vi "output.vi"(8 "error in":errorcluster, 10 "data table in":T1, 11 "EIP Tags Runtime in":refnum<class "EIP Tags Runtime.lvclass">) -> (0 "error out":errorcluster, 2 "data table out":T1, 3 "EIP Tags Runtime out":refnum<class "EIP Tags Runtime.lvclass">)   [LabVIEW 2013, in "EIP Tags Runtime.lvclass"]
doc: "Provides an interface for writing data to a module at runtime. While this interface performs no operations, a child should provide an override which may write to any open sessions, references, or interfaces."
uses:
  EIP Tags Runtime.lvclass
  <vilib>/NI/Tag Bus/table/data table.ctl
  EIP Tags Runtime.lvclass/EIP Tags Runtime.ctl
  <vilib>/NI/Tag Bus/table/data polymorphs/read many/read I8s.vi
  <vilib>/NI/Tag Bus/table/data polymorphs/read one/read Array of I8.vi
  <vilib>/NI/Tag Bus/table/data polymorphs/read many/read I16s.vi
  <vilib>/NI/Tag Bus/table/data polymorphs/read one/read Array of I16.vi
  <vilib>/NI/Tag Bus/table/data polymorphs/read many/read I32s.vi
  <vilib>/NI/Tag Bus/table/data polymorphs/read one/read Array of I32.vi
  <vilib>/NI/Tag Bus/table/data polymorphs/read many/read Singles.vi
  <vilib>/NI/Tag Bus/table/data polymorphs/read one/read Array of Single.vi
  <vilib>/NI/Tag Bus/table/data polymorphs/read many/read Booleans.vi
  <vilib>/NI/Tag Bus/table/data polymorphs/read one/read Array of Boolean.vi
  <vilib>/NI/Tag Bus/table/data polymorphs/read one/read String.vi
  <vilib>/ethernetip/ethernetip.llb/EthernetIP Tag Write SINT.vi
  <vilib>/ethernetip/ethernetip.llb/EthernetIP Tag Write INT.vi
  <vilib>/ethernetip/ethernetip.llb/EthernetIP Tag Write DINT.vi
  <vilib>/ethernetip/ethernetip.llb/EthernetIP Tag Write REAL.vi
  <vilib>/ethernetip/ethernetip.llb/EthernetIP Tag Write BOOL.vi
  <vilib>/ethernetip/ethernetip.llb/EthernetIP Tag Write STRING.vi
  <vilib>/NI/Tag Bus/table/data table.lvlib
  <vilib>/ethernetip/ethernetip.lvlib
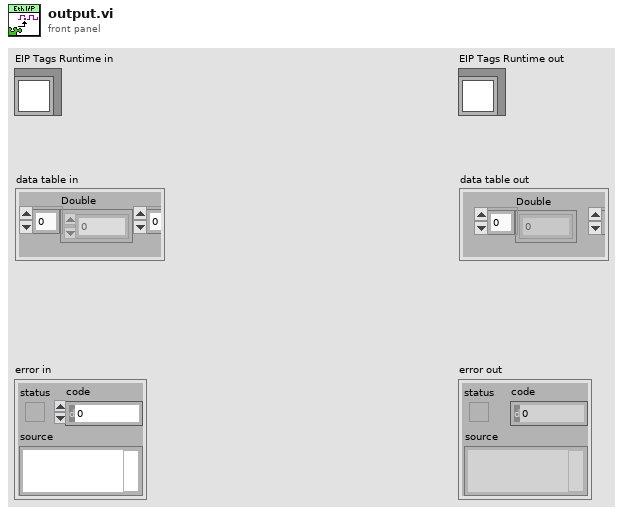
[diagram p1: front panel]
types:
  T1 = typedef "tag bus.lvlib/data table.lvlib/data table.ctl" = cluster{"Double":dbl[], "Single":sgl[], "I64":i64[], "I32":i32[], "I16":i16[], "I8":i8[], "U64":u64[], "U32":u32[], "U16":u16[], "U8":u8[], "Boolean":bool[], "String":string[], "Array of Double":cluster{"DBL Array":dbl[]}[], "Array of Single":cluster{"SGL Array":sgl[]}[], "Array of I64":cluster{"I64 Array":i64[]}[], "Array of I32":cluster{"I32 Array":i32[]}[], "Array of I16":cluster{"I16 Array":i16[]}[], "Array of I8":cluster{"I8 Array":i8[]}[], "Array of U64":cluster{"U64 Array":u64[]}[], "Array of U32":cluster{"U32 Array":u32[]}[], "Array of U16":cluster{"U16 Array":u16[]}[], "Array of U8":cluster{"U8 Array":u8[]}[], "Array of Boolean":cluster{"Boolean Array":bool[]}[], "Array of String":cluster{"String Array":string[]}[]}
  T2 = typedef "ethernetip.lvlib/ethernetip.ctl" = refnum<k21>
  T3 = typedef "EIP Tags Runtime.lvclass/eip tag spec.ctl" = cluster{"eip tag types":T4, "Network Path":string, "Tag Name":string, "Number of Elements":u32, "data indices":i32[], "tag bus indices":i32[], "array tbtag":bool}
  T4 = typedef "EIP Tags Configuration.lvclass/eip tag types.ctl" = enum16{"SINT", "INT", "DINT", "REAL", "BOOL", "STRING"}
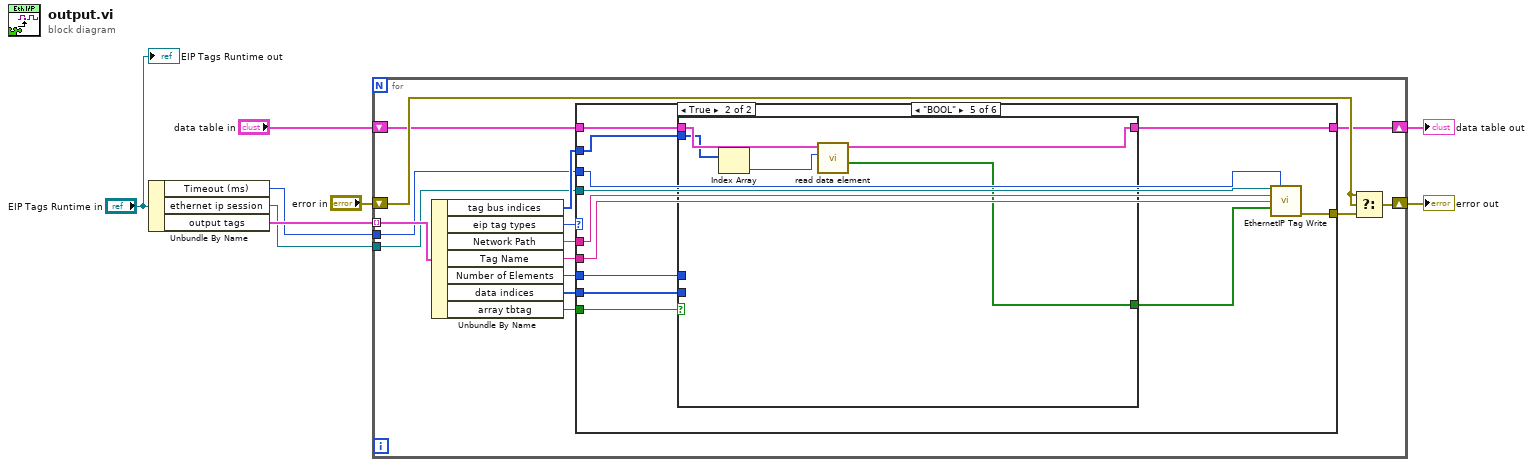
[diagram p0: block diagram]
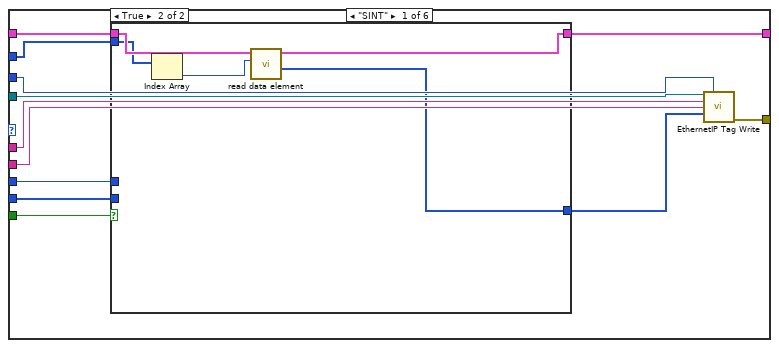
[diagram p2: hidden frame]
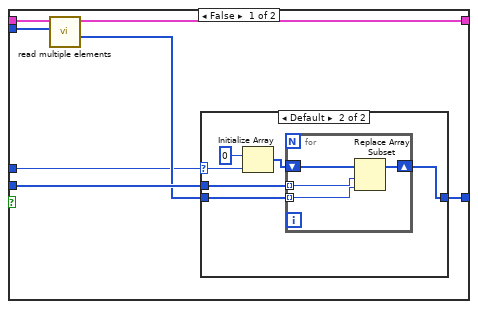
[diagram p3: hidden frame]
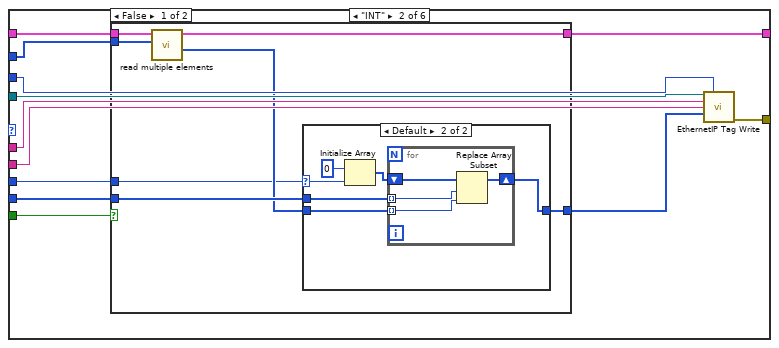
[diagram p5: hidden frame]
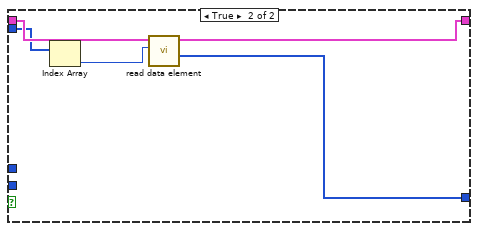
[diagram p7: hidden frame]
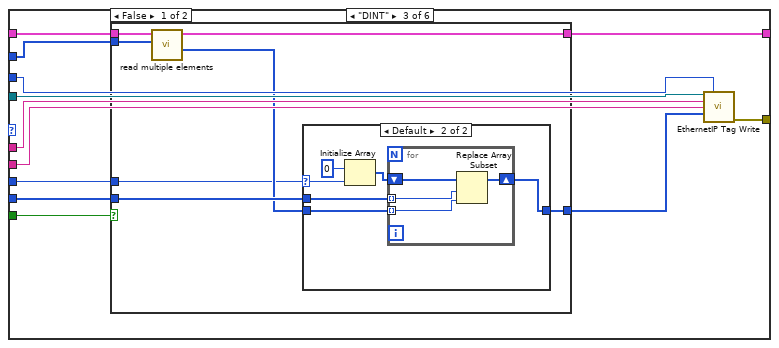
[diagram p8: hidden frame]
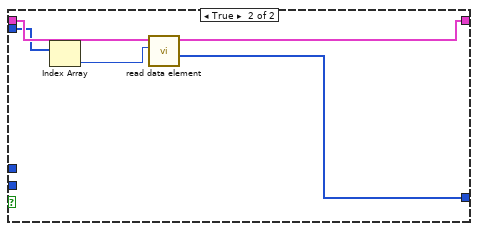
[diagram p10: hidden frame]
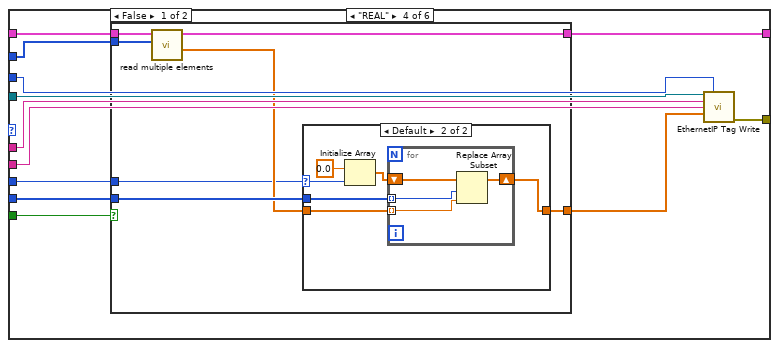
[diagram p11: hidden frame]
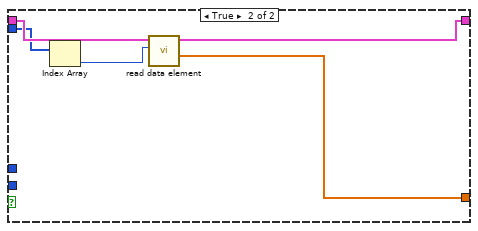
[diagram p13: hidden frame]
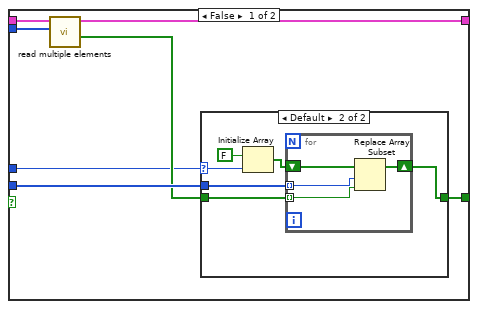
[diagram p14: hidden frame]
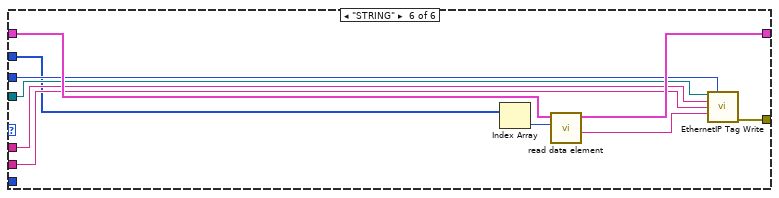
[diagram p16: hidden frame]
diagram:
  n1 = Unbundle By Name("EIP Tags Runtime in") -> ("Timeout (ms)"=w1:i32, "ethernet ip session"=w2:T2, "output tags"=w3:T3[])
  n2 = for {
    shift-right: [w22] -> w7
    shift-left: "error in" -> [w23]
    shift-right: [w19] -> w5
    shift-left: "data table in" -> [w18]
    tunnel: w3 -> [w21] mode=indexing
    tunnel: w2 -> [w16]
    tunnel: w1 -> [w15]
    n3 = Unbundle By Name(w21) -> ("tag bus indices"=w17:i32[], "eip tag types"=w20:T4, "Network Path"=w14:string, "Tag Name"=w13:string, "Number of Elements"=w12:u32, "data indices"=w10:i32[], "array tbtag"=w9:bool)
    n4 = case shown="\"BOOL\"" w20 {
      tunnel: [w34 w69 w104 w139 w174 w207] -> w19
      tunnel: w18 -> [w35 w70 w105 w140 w175 w208]
      tunnel: w17 -> [w33 w68 w103 w138 w173 w201]
      tunnel: w16 -> [w32 w67 w102 w137 w172 w206]
      tunnel: w15 -> [w31 w66 w101 w136 w171 w205]
      tunnel: w14 -> [w30 w65 w100 w135 w170 w204]
      tunnel: w13 -> [w29 w64 w99 w134 w169 w203]
      tunnel: w12 -> [w25 w60 w95 w130 w165 _]
      tunnel: [w27 w62 w97 w132 w167 w202] -> w11
      tunnel: w10 -> [w26 w61 w96 w131 w166 _]
      tunnel: w9 -> [w24 w59 w94 w129 w164 _]
      frame "SINT" {
        n5 = case shown="True" w24 {
          tunnel: w35 -> [w42 w58]
          tunnel: [w41 w54] -> w34
          tunnel: w33 -> [w40 w57]
          tunnel: [w39 w55] -> w28
          tunnel: w26 -> [w38 _]
          tunnel: w25 -> [w36 _]
          frame False {
            n6 = call-poly <vilib>:"read multiple elements.vi"("indices"=w40, "data table in"=w42) -> ("values"=w37:i8[], "data table out"=w41:T1)  [unwired: 8 in]
            n7 = case shown="Default" w36 {
              selector: w36 -> [_ w44]
              tunnel: [w43 w47] -> w39
              tunnel: w38 -> [_ w46]
              tunnel: w37 -> [w43 w45]
              frame 1 {
              }
              frame Default {
                n8 = Initialize Array(i8 0, w44) -> (w48:i8[])
                n9 = for {
                  shift-right: [w52] -> w47
                  shift-left: w48 -> [w53]
                  tunnel: w46 -> [w51] mode=indexing
                  tunnel: w45 -> [w50] mode=indexing
                  n10 = Replace Array Subset(array=w53, new element=w50, index=w51) -> (w52:i8[])
                }
              }
            }
          }
          frame True {
            n11 = Index Array(array=w57) -> (element=w56:i32)  [unwired: 1 in]
            n12 = call-poly <vilib>:"read data element.vi"("index"=w56, "data table in"=w58) -> ("value"=w55:i8[], "data table out"=w54:T1)  [unwired: 8 in]
          }
        }
        n13 = call-poly <vilib>:"EthernetIP Tag Write.vi"("Session in"=w32, "Timeout (ms)"=w31, "Network Path"=w30, "Tag Name"=w29, "Data"=w28) -> ("error out"=w27:errorcluster)  [unwired: 9 in, 1 out]
      }
      frame "INT" {
        n14 = case shown="False" w59 {
          tunnel: w70 -> [w77 w93]
          tunnel: [w76 w89] -> w69
          tunnel: w68 -> [w75 w92]
          tunnel: [w74 w90] -> w63
          tunnel: w61 -> [w73 _]
          tunnel: w60 -> [w71 _]
          frame False {
            n15 = call-poly <vilib>:"read multiple elements.vi"("indices"=w75, "data table in"=w77) -> ("values"=w72:i16[], "data table out"=w76:T1)  [unwired: 8 in]
            n16 = case shown="Default" w71 {
              selector: w71 -> [_ w79]
              tunnel: [w78 w82] -> w74
              tunnel: w73 -> [_ w81]
              tunnel: w72 -> [w78 w80]
              frame 1 {
              }
              frame Default {
                n17 = Initialize Array(i16 0, w79) -> (w83:i16[])
                n18 = for {
                  shift-right: [w87] -> w82
                  shift-left: w83 -> [w88]
                  tunnel: w81 -> [w86] mode=indexing
                  tunnel: w80 -> [w85] mode=indexing
                  n19 = Replace Array Subset(array=w88, new element=w85, index=w86) -> (w87:i16[])
                }
              }
            }
          }
          frame True {
            n20 = Index Array(array=w92) -> (element=w91:i32)  [unwired: 1 in]
            n21 = call-poly <vilib>:"read data element.vi"("index"=w91, "data table in"=w93) -> ("value"=w90:i16[], "data table out"=w89:T1)  [unwired: 8 in]
          }
        }
        n22 = call-poly <vilib>:"EthernetIP Tag Write.vi"("Session in"=w67, "Timeout (ms)"=w66, "Network Path"=w65, "Tag Name"=w64, "Data"=w63) -> ("error out"=w62:errorcluster)  [unwired: 9 in, 1 out]
      }
      frame "DINT" {
        n23 = case shown="False" w94 {
          tunnel: w105 -> [w112 w128]
          tunnel: [w111 w124] -> w104
          tunnel: w103 -> [w110 w127]
          tunnel: [w109 w125] -> w98
          tunnel: w96 -> [w108 _]
          tunnel: w95 -> [w106 _]
          frame False {
            n24 = call-poly <vilib>:"read multiple elements.vi"("indices"=w110, "data table in"=w112) -> ("values"=w107:i32[], "data table out"=w111:T1)  [unwired: 8 in]
            n25 = case shown="Default" w106 {
              selector: w106 -> [_ w114]
              tunnel: [w113 w117] -> w109
              tunnel: w108 -> [_ w116]
              tunnel: w107 -> [w113 w115]
              frame 1 {
              }
              frame Default {
                n26 = Initialize Array(0, w114) -> (w118:i32[])
                n27 = for {
                  shift-right: [w122] -> w117
                  shift-left: w118 -> [w123]
                  tunnel: w116 -> [w121] mode=indexing
                  tunnel: w115 -> [w120] mode=indexing
                  n28 = Replace Array Subset(array=w123, new element=w120, index=w121) -> (w122:i32[])
                }
              }
            }
          }
          frame True {
            n29 = Index Array(array=w127) -> (element=w126:i32)  [unwired: 1 in]
            n30 = call-poly <vilib>:"read data element.vi"("index"=w126, "data table in"=w128) -> ("value"=w125:i32[], "data table out"=w124:T1)  [unwired: 8 in]
          }
        }
        n31 = call-poly <vilib>:"EthernetIP Tag Write.vi"("Session in"=w102, "Timeout (ms)"=w101, "Network Path"=w100, "Tag Name"=w99, "Data"=w98) -> ("error out"=w97:errorcluster)  [unwired: 9 in, 1 out]
      }
      frame "REAL" {
        n32 = case shown="False" w129 {
          tunnel: w140 -> [w147 w163]
          tunnel: [w146 w159] -> w139
          tunnel: w138 -> [w145 w162]
          tunnel: [w144 w160] -> w133
          tunnel: w131 -> [w143 _]
          tunnel: w130 -> [w141 _]
          frame False {
            n33 = call-poly <vilib>:"read multiple elements.vi"("indices"=w145, "data table in"=w147) -> ("values"=w142:sgl[], "data table out"=w146:T1)  [unwired: 8 in]
            n34 = case shown="Default" w141 {
              selector: w141 -> [_ w149]
              tunnel: [w148 w152] -> w144
              tunnel: w143 -> [_ w151]
              tunnel: w142 -> [w148 w150]
              frame 1 {
              }
              frame Default {
                n35 = Initialize Array(sgl 0.0, w149) -> (w153:sgl[])
                n36 = for {
                  shift-right: [w157] -> w152
                  shift-left: w153 -> [w158]
                  tunnel: w151 -> [w156] mode=indexing
                  tunnel: w150 -> [w155] mode=indexing
                  n37 = Replace Array Subset(array=w158, new element=w155, index=w156) -> (w157:sgl[])
                }
              }
            }
          }
          frame True {
            n38 = Index Array(array=w162) -> (element=w161:i32)  [unwired: 1 in]
            n39 = call-poly <vilib>:"read data element.vi"("index"=w161, "data table in"=w163) -> ("value"=w160:sgl[], "data table out"=w159:T1)  [unwired: 8 in]
          }
        }
        n40 = call-poly <vilib>:"EthernetIP Tag Write.vi"("Session in"=w137, "Timeout (ms)"=w136, "Network Path"=w135, "Tag Name"=w134, "Data"=w133) -> ("error out"=w132:errorcluster)  [unwired: 9 in, 1 out]
      }
      frame "BOOL" {
        n41 = case shown="True" w164 {
          tunnel: w175 -> [w182 w198]
          tunnel: [w181 w194] -> w174
          tunnel: w173 -> [w180 w197]
          tunnel: [w179 w195] -> w168
          tunnel: w166 -> [w178 _]
          tunnel: w165 -> [w176 _]
          frame False {
            n42 = call-poly <vilib>:"read multiple elements.vi"("indices"=w180, "data table in"=w182) -> ("values"=w177:bool[], "data table out"=w181:T1)  [unwired: 8 in]
            n43 = case shown="Default" w176 {
              selector: w176 -> [_ w184]
              tunnel: [w183 w187] -> w179
              tunnel: w178 -> [_ w186]
              tunnel: w177 -> [w183 w185]
              frame 1 {
              }
              frame Default {
                n44 = Initialize Array(FALSE, w184) -> (w188:bool[])
                n45 = for {
                  shift-right: [w192] -> w187
                  shift-left: w188 -> [w193]
                  tunnel: w186 -> [w191] mode=indexing
                  tunnel: w185 -> [w190] mode=indexing
                  n46 = Replace Array Subset(array=w193, new element=w190, index=w191) -> (w192:bool[])
                }
              }
            }
          }
          frame True {
            n47 = Index Array(array=w197) -> (element=w196:i32)  [unwired: 1 in]
            n48 = call-poly <vilib>:"read data element.vi"("index"=w196, "data table in"=w198) -> ("value"=w195:bool[], "data table out"=w194:T1)  [unwired: 8 in]
          }
        }
        n49 = call-poly <vilib>:"EthernetIP Tag Write.vi"("Session in"=w172, "Timeout (ms)"=w171, "Network Path"=w170, "Tag Name"=w169, "Data"=w168) -> ("error out"=w167:errorcluster)  [unwired: 9 in, 1 out]
      }
      frame "STRING" {
        n50 = Index Array(array=w201) -> (element=w200:i32)  [unwired: 1 in]
        n51 = call-poly <vilib>:"read data element.vi"("index"=w200, "data table in"=w208) -> ("value"=w199:string, "data table out"=w207:T1)  [unwired: 8 in]
        n52 = call-poly <vilib>:"EthernetIP Tag Write.vi"("Session in"=w206, "Timeout (ms)"=w205, "Network Path"=w204, "Tag Name"=w203, "Data"=w199) -> ("error out"=w202:errorcluster)  [unwired: 9 in, 1 out]
      }
    }
    n53 = Select(t=w23, s=w23, f=w11) -> (s? t:f=w22:errorcluster)
  }
  "error out" <- w7
  "data table out" <- w5
  "EIP Tags Runtime out" <- "EIP Tags Runtime in"
